vi "VIE.Module.Queued Message Handler.flush.QueuedMessageHandler.vi"(8 "error in (no error)":errorcluster, 10 "QueuedMessageHandler.dqGOOPClass (in)":T1) -> (0 "error out":errorcluster, 1 "States Flushed":string[](array[string]), 2 "QueuedMessageHandler.dqGOOPClass (out)":T1)   [LabVIEW 2010, in "VIE.Module.Queued Message Handler.QueuedMessageHandler.dqGOOPClass.lvlib"]
uses:
  VIE.Module.Queued Message Handler.QueuedMessageHandler.dqGOOPClass.lvlib
  VIE.Module.Queued Message Handler.dqClass_ObjectReference.ctl
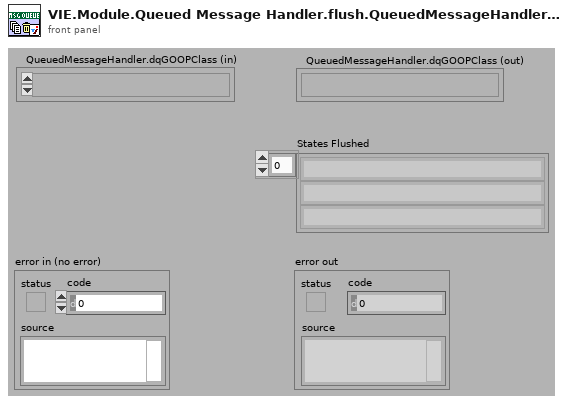
[diagram p1: front panel]
types:
  T1 = typedef "VIE.Module.Queued Message Handler.QueuedMessageHandler.dqGOOPClass.lvlib/VIE.Module.Queued Message Handler.dqClass_ObjectReference.ctl" = refnum<k1>
  T2 = typedef "VIE.Module.Queued Message Handler.QueuedMessageHandler.dqGOOPClass.lvlib/VIE.Module.Queued Message Handler.dqClass_ObjectData.ctl" = cluster{"Message Queue":refnum<queue>, "Log File Refnum":refnum<file>}
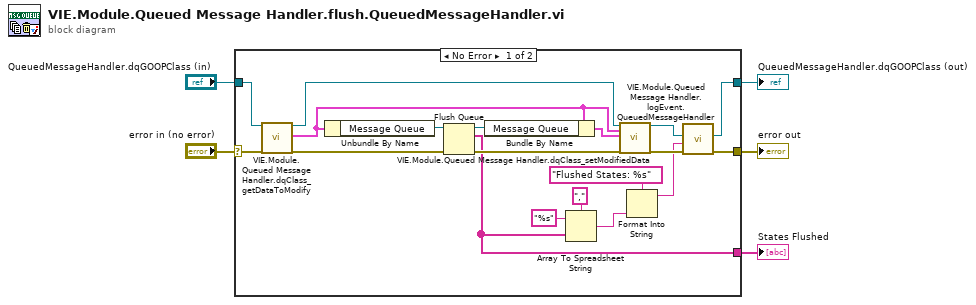
[diagram p0: block diagram]
diagram:
  n1 = case shown="No Error" "error in (no error)" {
    selector: "error in (no error)" -> [w22 w26]
    tunnel: [w10 w26] -> w4
    tunnel: [w6 w25] -> w3
    tunnel: "QueuedMessageHandler.dqGOOPClass (in)" -> [w20 w25]
    tunnel: [w8 _] -> w1
    frame No Error {
      n2 = call "VIE.Module.Queued Message Handler.dqClass_getDataToModify.vi"("reference"=w20, "error in (no error)"=w22) -> ("duplicate reference"=w19:T1, "data"=w18:T2, "error out"=w21:errorcluster)  [unwired: 14 in, 1 out]
      n3 = Unbundle By Name(w18) -> ("Message Queue"=w24:refnum<queue>)
      n4 = Flush Queue(queue=w24, error in (no error)=w21) -> (queue out=w23:refnum<queue>, remaining elements=w8:string[], error out=w12:errorcluster)
      n5 = Bundle By Name(cluster=w18, "Message Queue"=w23) -> (w17:T2)
      n6 = Array To Spreadsheet String(delimiter (Tab)=",", array=w8, 3:"%s" ("format string")) -> (spreadsheet string=w13:string)
      n7 = call "VIE.Module.Queued Message Handler.dqClass_setModifiedData.vi"("reference"=w19, "data (unmodified)"=w18, "data"=w17, "error in (no error)"=w12) -> ("duplicate reference"=w9:T1, "error out"=w11:errorcluster)  [unwired: 14 in]
      n8 = Format Into String(format string="Flushed States: %s", w13) -> (resulting string=w7:string)  [unwired: 2 in, 1 out]
      n9 = call "VIE.Module.Queued Message Handler.logEvent.QueuedMessageHandler.vi"("error in (no error)"=w11, "Event to Log"=w7, "QueuedMessageHandler.dqGOOPClass (in)"=w9) -> ("error out"=w10:errorcluster, "QueuedMessageHandler.dqGOOPClass (out)"=w6:T1)  [unwired: 7 in]
    }
    frame Error {
    }
  }
  "error out" <- w4
  "QueuedMessageHandler.dqGOOPClass (out)" <- w3
  "States Flushed" <- w1
